vi "FixedTrigger.vi"(8 "array in":bool[](array[boolean])=[FALSE, FALSE, FALSE, FALSE, FALSE, FALSE, FALSE, FALSE, FALSE], 9 "IO Module\\Synchronous Trigger Input":u8, 11 "Last? Input":bool) -> (0 "array out":bool[](array[boolean]), 1 "trigger out":bool[](array[boolean]))   [LabVIEW 2012]
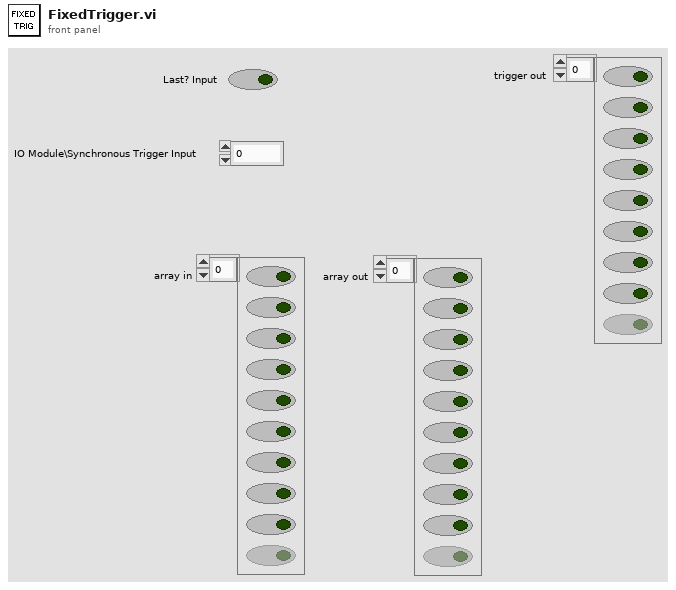
[diagram p1: front panel]
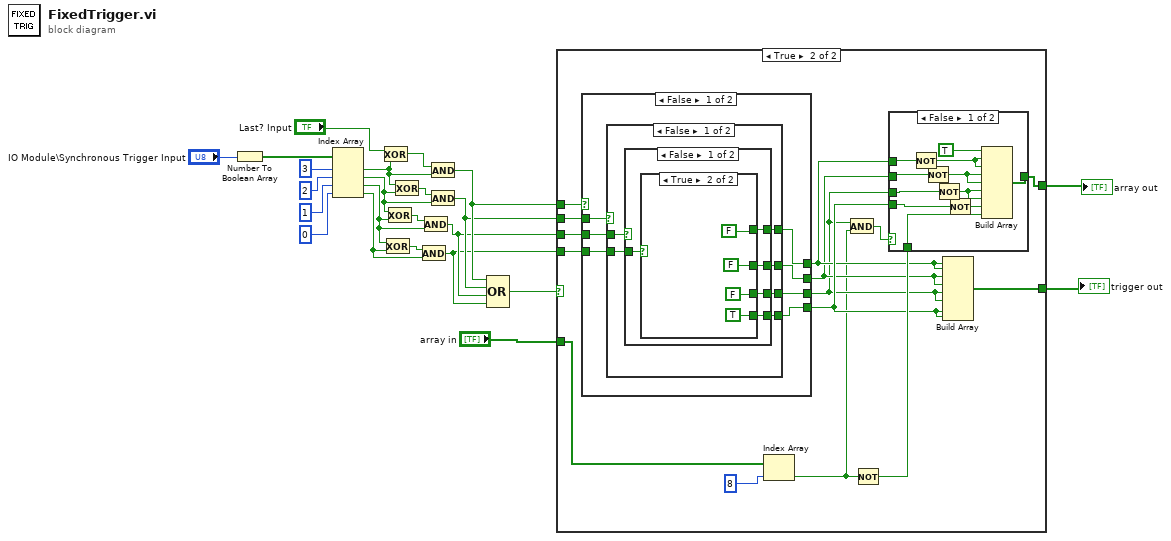
[diagram p0: block diagram]
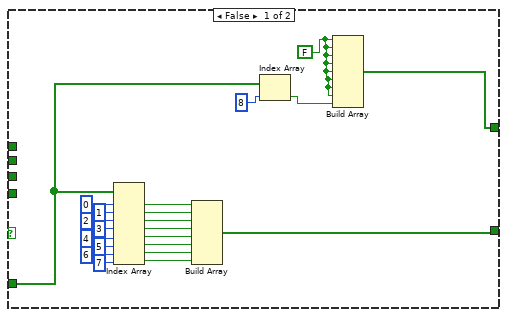
[diagram p2: hidden frame]
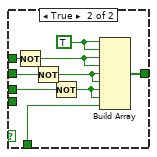
[diagram p3: hidden frame]
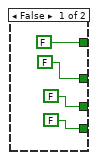
[diagram p4: hidden frame]
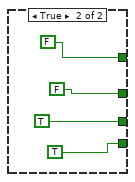
[diagram p5: hidden frame]
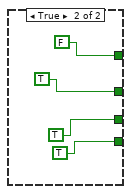
[diagram p6: hidden frame]
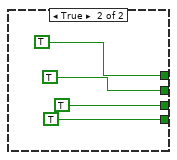
[diagram p7: hidden frame]
diagram:
  n1 = Number To Boolean Array(number="IO Module\\Synchronous Trigger Input") -> (Boolean array=w23:bool[])
  n2 = Index Array(array=w23, index #1=3, index #2=2, index #3=1, index #4=0) -> (element #1=w17:bool, element #2=w15:bool, element #3=w13:bool, element #4=w12:bool)
  n3 = Exclusive Or(1:w17, 2:"Last? Input") -> (0:w18:bool)
  n4 = Exclusive Or(1:w12, 2:w13) -> (0:w11:bool)
  n5 = Exclusive Or(1:w13, 2:w15) -> (0:w14:bool)
  n6 = Exclusive Or(1:w15, 2:w17) -> (0:w16:bool)
  n7 = And(x=w11, y=w12) -> (x .and. y?=w7:bool)
  n8 = And(x=w14, y=w13) -> (x .and. y?=w8:bool)
  n9 = And(x=w18, y=w17) -> (x .and. y?=w10:bool)
  n10 = And(x=w16, y=w15) -> (x .and. y?=w9:bool)
  n11 = Compound Arithmetic op=OR(w10, w9, w8, w7) -> (w6:bool)
  n12 = case shown="True" w6 {
    tunnel: w10 -> [_ w60]
    tunnel: w9 -> [_ w59]
    tunnel: w8 -> [_ w58]
    tunnel: w7 -> [_ w55]
    tunnel: "array in" -> [w26 w53]
    tunnel: [w37 w57] -> w2
    tunnel: [w27 w56] -> w3
    frame False {
      w25 = FALSE
      n13 = Index Array(array=w26, index #1=0 ("index"), index #2=1 ("index"), index #3=2 ("index"), index #4=3 ("index"), index #5=4 ("index"), index #6=5 ("index"), index #7=6 ("index"), index #8=7 ("index")) -> (element #1=w38:bool, element #2=w45:bool, element #3=w44:bool, element #4=w43:bool, element #5=w42:bool, element #6=w41:bool, element #7=w40:bool, element #8=w39:bool)
      n14 = Build Array(w38, w45, w44, w43, w42, w41, w40, w39) -> (w37:bool[])
      n15 = Index Array(array=w26, index=8) -> (element=w24:bool)
      n16 = Build Array(w25, w25, w25, w25, w25, w25, w25, w25, w24) -> (w27:bool[])
    }
    frame True {
      n17 = case shown="False" w60 {
        tunnel: w59 -> [w87 _]
        tunnel: w58 -> [w86 _]
        tunnel: w55 -> [w85 _]
        tunnel: [w82 TRUE] -> w50
        tunnel: [w83 TRUE] -> w49
        tunnel: [w84 TRUE] -> w48
        tunnel: [w81 TRUE] -> w51
        frame False {
          n18 = case shown="False" w87 {
            tunnel: w86 -> [w93 _]
            tunnel: w85 -> [w92 _]
            tunnel: [w91 TRUE] -> w81
            tunnel: [w90 TRUE] -> w84
            tunnel: [w89 TRUE] -> w83
            tunnel: [w88 FALSE] -> w82
            frame False {
              n19 = case shown="False" w93 {
                tunnel: w92 -> [w98 _]
                tunnel: [w97 TRUE] -> w91
                tunnel: [w96 TRUE] -> w90
                tunnel: [w95 FALSE] -> w89
                tunnel: [w94 FALSE] -> w88
                frame False {
                  n20 = case shown="True" w98 {
                    tunnel: [FALSE TRUE] -> w97
                    tunnel: [FALSE FALSE] -> w96
                    tunnel: [FALSE FALSE] -> w95
                    tunnel: [FALSE FALSE] -> w94
                    frame False {
                    }
                    frame True {
                    }
                  }
                }
                frame True {
                }
              }
            }
            frame True {
            }
          }
        }
        frame True {
        }
      }
      n21 = Index Array(array=w53, index=8) -> (element=w47:bool)
      n22 = And(x=w48, y=w47) -> (x .and. y?=w46:bool)
      n23 = Not(x=w47) -> (.not. x?=w52:bool)
      n24 = case shown="False" w46 {
        tunnel: w50 -> [w71 w80]
        tunnel: w49 -> [w70 w79]
        tunnel: w48 -> [w66 w78]
        tunnel: [w69 w77] -> w56
        tunnel: w52 -> [w67 w72]
        tunnel: w51 -> [w62 _]
        frame False {
          n25 = Not(x=w71) -> (.not. x?=w65:bool)
          n26 = Not(x=w70) -> (.not. x?=w64:bool)
          n27 = Not(x=w66) -> (.not. x?=w63:bool)
          n28 = Not(x=w62) -> (.not. x?=w61:bool)
          n29 = Build Array(TRUE, w65, w65, w64, w64, w63, w63, w61, w67) -> (w69:bool[])
        }
        frame True {
          w76 = TRUE
          n30 = Not(x=w80) -> (.not. x?=w75:bool)
          n31 = Not(x=w79) -> (.not. x?=w74:bool)
          n32 = Not(x=w78) -> (.not. x?=w73:bool)
          n33 = Build Array(w76, w76, w75, w75, w74, w74, w73, w73, w72) -> (w77:bool[])
        }
      }
      n34 = Build Array(w50, w50, w49, w49, w48, w48, w51, w51) -> (w57:bool[])
    }
  }
  "array out" <- w3
  "trigger out" <- w2
